vi "ChooseDirection.vi"(1 "UseLV2011Compatibility":bool, 2 "IsErrorCluster":bool, 3 "ISOutput":bool) -> (0 "Dir 2":T1=enum."Output")   [LabVIEW 2020]
uses:
  <vilib>/AppBuilder/IOStatus.ctl
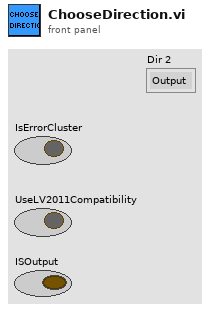
[diagram p1: front panel]
types:
  T1 = typedef "IOStatus.ctl" = enum16{"Input", "Output", "Input/Output", "InputDeleted", "OutputDeleted", "IODeleted", "ErrorClusterIn", "ErrorClusterOut"}
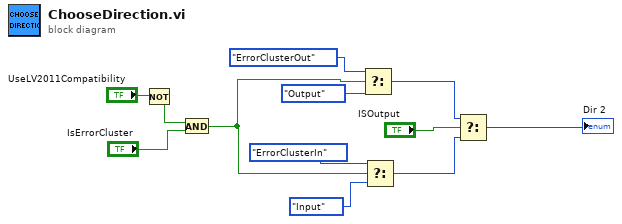
[diagram p0: block diagram]
diagram:
  n1 = Not(x="UseLV2011Compatibility") -> (.not. x?=w11:bool)
  n2 = And(x=w11, y="IsErrorCluster") -> (x .and. y?=w2:bool)
  n3 = Select(t=IOStatus."ErrorClusterOut" ("Dir"), s=w2, f=IOStatus."Output" ("Input/Output")) -> (s? t:f=w9:T1)
  n4 = Select(t=IOStatus."ErrorClusterIn" ("Input/Output"), s=w2, f=IOStatus."Input" ("Dir")) -> (s? t:f=w8:T1)
  n5 = Select(t=w9, s="ISOutput", f=w8) -> (s? t:f=→"Dir 2":T1)
